vi "New VIEventHandler.vi"(6 "EventFilter Reference":T1, 7 "Timeout Message Priority (Normal)":T2=enum."Normal", 8 "Timeout [ms]":i32=-1, 9 "Timeout Message":refnum<class "Message.lvclass">, 10 "Registrations":T3[](array[typedef]), 11 "VI Refnum":refnum<vi>) -> (0 "error out":errorcluster, 3 "VIEventHandler":refnum<class "VIEventHandler.lvclass">)   [LabVIEW 2019, in "ActorEvents.lvlib" / "VIEventHandler.lvclass"]
uses:
  <vilib>/gpm_packages/@cs/mva-viewable/Source/ActorEvents/EventHandler/VIEventHandler/VIEventHandler.lvclass
  C:/Program Files/National Instruments/LabVIEW 2019/vi.lib/gpm_packages/@cs/mva-viewable/Source/ActorEvents/IEventHandler/IEventHandler.lvclass
  <vilib>/event_ctls.llb/lveventtype.ctl
  <vilib>/ActorFramework/Message/Message.lvclass
  <vilib>/ActorFramework/Message Enqueuer/Message Priority.ctl
  <vilib>/gpm_packages/@cs/mva-viewable/Source/ActorEvents/IEventFilter/EventFilter Reference.ctl
  <vilib>/gpm_packages/@cs/mva-viewable/Source/ActorEvents/IEventFilter/IEventFilter.lvclass
  <vilib>/gpm_packages/@cs/mva-viewable/Source/ActorEvents/IEventHandler/IEventHandler.lvclass/IEventHandler.ctl
  <vilib>/gpm_packages/@cs/mva-viewable/Source/ActorEvents/EventHandler/VIEventHandler/VIEventHandler.lvclass/VIEventHandler.ctl
  <vilib>/Utility/error.llb/Error Cluster From Error Code.vi
  <vilib>/gpm_packages/@cs/mva-viewable/Source/ActorEvents/IEventHandler/IEventHandler.lvclass
  <vilib>/ActorFramework/Message Enqueuer/Message Enqueuer.lvclass
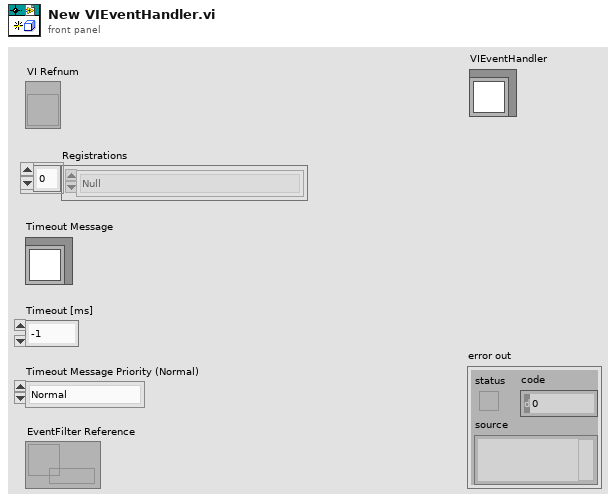
[diagram p1: front panel]
types:
  T1 = typedef "ActorEvents.lvlib/IEventFilter.lvclass/EventFilter Reference.ctl" = refnum<data-value>
  T2 = typedef "Actor Framework.lvlib/Message Enqueuer.lvclass/Message Priority.ctl" = enum16{"Low", "Normal", "High"}
  T3 = typedef "lveventtype.ctl" = enum32{"Null", "Timeout", "Annotation Menu Selection", "Annotation Menu Selection?", "App Instance Close", "App Instance Close?", "Autoscale Range Change", "Bookmark Info Change", "Cell Edit", "Cell Edit?", "Cursor Grab", "Cursor Grab?", "Cursor Menu Selection", "Cursor Menu Selection?", "Cursor Move", "Cursor Release", "Data Change", "Direction Change", "Display State Change", "Drag Ended", "Drag Enter", "Drag Leave", "Drag Over", "Drag Source Update", "Drag Starting", "Drag Starting?", "Drop", "Exec State Change", "Key Down", "Key Down?", "Key Repeat", "Key Repeat?", "Key Up", "Listbox Double Click", "Menu Activation?", "Menu Selection (App)", "Menu Selection? (App)", "Menu Selection (User)", "Mouse Down", "Mouse Down?", "Mouse Enter", "Mouse Leave", "Mouse Move", "Mouse Up", "Mouse Wheel", "NI Security User Change (App)", "Pane Size", "Panel Close", "Panel Close?", "Panel Resize", "Plot Attribute Change", "Scale Range Change", "Shortcut Menu Activation?", "Shortcut Menu Selection (App)", "Shortcut Menu Selection? (App)", "Shortcut Menu Selection (User)", "Tree Double Click", "Tree Drag", "Tree Drag?", "Tree Drop", "Tree Drop?", "Tree Item Close", "Tree Item Close?", "Tree Item Open", "Tree Item Open?", "User Event", "Value Change"}
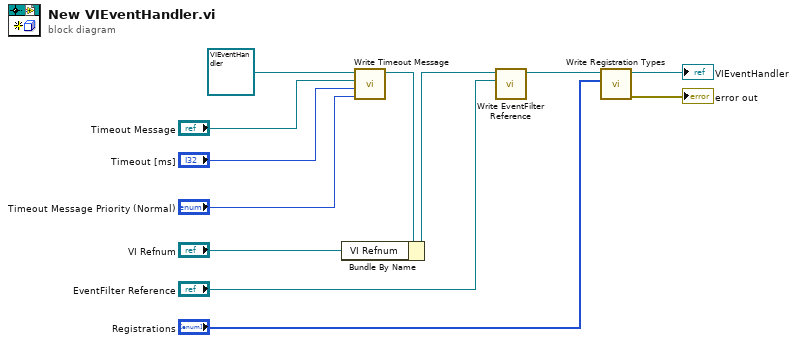
[diagram p0: block diagram]
diagram:
  n1 = call <vilib>:"Write Timeout Message.vi"("Timeout Message Priority (Normal)"="Timeout Message Priority (Normal)", "Timeout [ms]"="Timeout [ms]", "Timeout Message"="Timeout Message", "IEventHandler in"=refnum<class "VIEventHandler.lvclass"> refnum ("VIEventHandler In")) -> ("IEventHandler out"=w11:refnum<class "VIEventHandler.lvclass">)  [unwired: 7 in]
  n2 = Bundle By Name(cluster=w11, "VI Refnum"="VI Refnum") -> (w12:refnum<class "VIEventHandler.lvclass">)
  n3 = call <vilib>:"Write EventFilter Reference.vi"("EventFilter Reference"="EventFilter Reference", "IEventHandler in"=w12) -> ("IEventHandler out"=w2:refnum<class "VIEventHandler.lvclass">)  [unwired: 9 in]
  n4 = call <vilib>:"Write Registration Types.vi"("Requested Registration Types"="Registrations", "IEventHandler In"=w2) -> ("error out"=→"error out":errorcluster, "IEventHandler Out"=→"VIEventHandler":refnum<class "VIEventHandler.lvclass">)  [unwired: 8 in]
